vi "GEA2 Serial Generate Command.vi"(8 "Error In":errorcluster, 9 "Xtra Command Data":u8[](array[numeric]), 10 "CMD Array":u8[](array[numeric]), 11 "Source Destination":T1 {"Destination" format="%x"; "Source" format="%x"}) -> (0 "Error Out":errorcluster, 2 "Byte Count":u32, 3 "Message Out":u8[](array[numeric]))   [LabVIEW 2014]
uses:
  Type Definitions/Source Destination Control.ctl
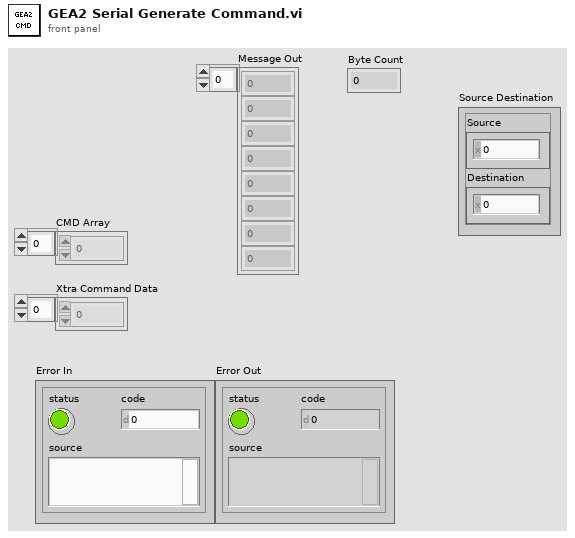
[diagram p1: front panel]
types:
  T1 = typedef "Source Destination Control.ctl" = cluster{"Source":u8, "Destination":u8}
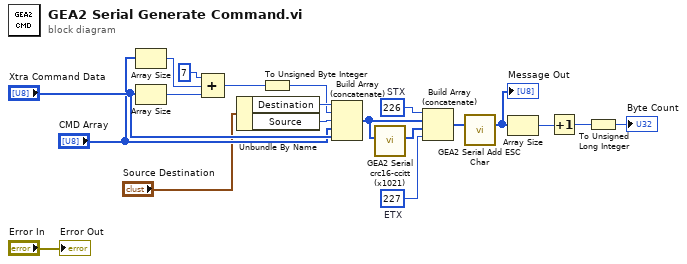
[diagram p0: block diagram]
diagram:
  w17 = u8 227  # ETX
  w14 = u8 226  # STX
  n1 = Array Size(array="CMD Array") -> (size(s)=w7:i32)
  n2 = Array Size(array="Xtra Command Data") -> (size(s)=w9:i32)
  n3 = Compound Arithmetic op=ADD(7 ("x"), w7, w9) -> (w11:i32)
  n4 = Unbundle By Name("Source Destination") -> ("Destination"=w19:u8, "Source"=w20:u8)
  n5 = To Unsigned Byte Integer(number=w11) -> (unsigned 8bit integer=w10:u8)
  n6 = Build Array (concatenate)(w19, w10, w20, "CMD Array", "Xtra Command Data") -> (w15:u8[])
  n7 = call "GEA2 Serial crc16-ccitt (x1021).vi"("unsigned byte array"=w15) -> ("CRC"=w16:u8[])  [unwired: 9 in, 1 out]
  n8 = Build Array (concatenate)(w14, w15, w16, w17) -> (w18:u8[])
  n9 = call "GEA2 Serial Add ESC Char.vi"("Message"=w18) -> ("Message Out"=w5:u8[])  [unwired: 14 in]
  "Message Out" <- w5
  n10 = Array Size(array=w5) -> (size(s)=w6:i32)
  n11 = Increment(x=w6) -> (x+1=w4:i32)
  n12 = To Unsigned Long Integer(number=w4) -> (unsigned 32bit integer=→"Byte Count":u32)
  "Error Out" <- "Error In"
